vi "Stop Teststand and Complete Sequence.vi"(7 "Stop Button":bool, 11 "SequenceContext":refnum<k7>) -> (0 "Error Out":errorcluster, 3 "Stop Button Out":bool)   [LabVIEW 2013]
doc: "This VI loops until either the Stop button is pressed or the calling TestStand sequence is terminated. The Termination Monitor VI allows this VI to query the TestStand execution for its current status.\n\nOnce the Stop button is pressed a output can be sued to update a variable in teststand"
uses:
  <vilib>/addons/TestStand/_TSUtility.llb/TestStand - Get Property Value (Boolean).vi
panel:
  # "This VI loops until either the Stop button is pressed or the calling TestStand sequence is terminated. The Termination Monitor VI allows this VI to query the TestStand execution for its current status."
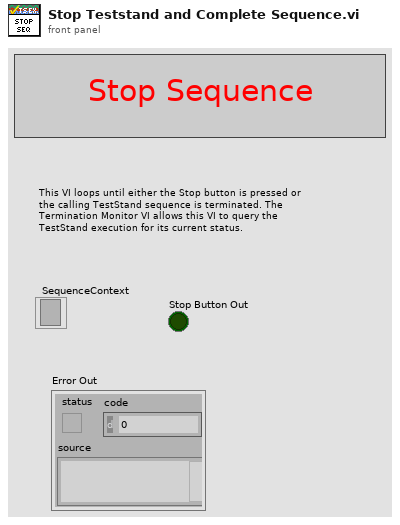
[diagram p1: front panel]
types:
  T1 = typedef "TestStand - Status Monitor.ctl" = cluster{"Sequence Context":refnum<k7>, "Execution":refnum<k7>, "Termination Monitor":refnum<k7>}
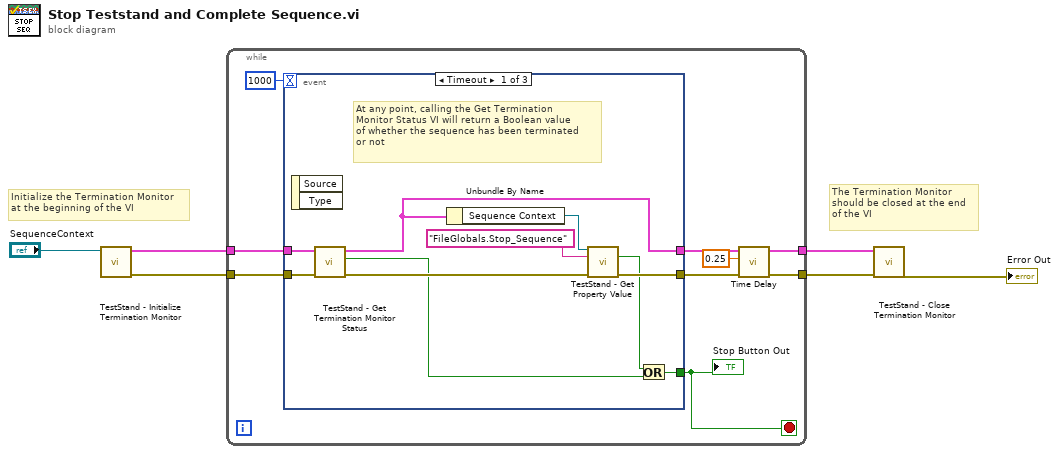
[diagram p0: block diagram]
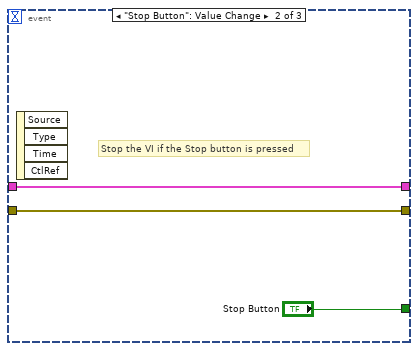
[diagram p2: hidden frame]
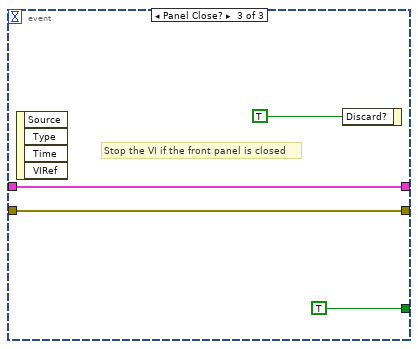
[diagram p3: hidden frame]
diagram:
  # "The Termination Monitor\nshould be closed at the end\nof the VI"
  # "Initialize the Termination Monitor\nat the beginning of the VI"
  n1 = call <vilib>:"TestStand - Initialize Termination Monitor.vi"("Sequence Context In"="SequenceContext") -> ("error out"=w1:errorcluster, "Status Monitor Out"=w5:T1)  [unwired: 9 in]
  n2 = while {
    tunnel: w5 -> [w13]
    tunnel: w1 -> [w12]
    tunnel: [w8] -> w4
    tunnel: [w11] -> w3
    stop <- w10 stop-if-true
    n3 = event shown="[0] Timeout" {
      selector: _ -> [_ _ _]
      dyn-events: _ -> [_ _ _]
      timeout: 1000 -> [_ _ _]
      tunnel: w13 -> [w24 w26 w30]
      tunnel: w12 -> [w23 w25 w29]
      tunnel: [w22 w25 w29] -> w9
      tunnel: [w21 w26 w30] -> w11
      tunnel: [w17 "Stop Button" TRUE ("Stop Button")] -> w10
      event Timeout {
        # "At any point, calling the Get Termination\nMonitor Status VI will return a Boolean value\nof whether the sequence has been terminated \nor not"
        n4 = event-data() -> ()  [unwired: 1 in, 2 out]
        n5 = call <vilib>:"TestStand - Get Termination Monitor Status.vi"("error in (no error)"=w23, "Status Monitor In"=w24) -> ("error out"=w19:errorcluster, "Terminating or Aborting"=w18:bool, "Status Monitor Out"=w21:T1)  [unwired: 7 in]
        n6 = Unbundle By Name(w21) -> ("Sequence Context"=w20:refnum<k7>)
        n7 = call-poly <vilib>:"TestStand - Get Property Value.vi"("Sequence Context In"=w20, "Lookup String"="FileGlobals.Stop_Sequence", "error in (no error)"=w19) -> ("Value"=w16:bool, "error out"=w22:errorcluster)  [unwired: 10 in, 1 out]
        n8 = Or(x=w16, y=w18) -> (x .or. y?=w17:bool)
      }
      event "Stop Button": Value Change {
        # "Stop the VI if the Stop button is pressed"
        n9 = event-data() -> ()  [unwired: 1 in, 4 out]
      }
      event Panel Close? {
        # "Stop the VI if the front panel is closed"
        n10 = event-data() -> ()  [unwired: 1 in, 4 out]
        n11 = event-data("Discard?"=TRUE) -> ()  [unwired: 1 in, 1 out]
      }
    }
    "Stop Button Out" <- w10
    n12 = call "Time Delay"("error in (no error)"=w9, "Delay Time (s)"=0.25) -> ("error out"=w8:errorcluster)  [unwired: 9 in]
  }
  n13 = call <vilib>:"TestStand - Close Termination Monitor.vi"("error in (no error)"=w4, "Status Monitor In"=w3) -> ("error out"=→"Error Out":errorcluster)  [unwired: 9 in]
